vi "MPB_JSON_step editor.vi"() -> ()   [LabVIEW 2020]
uses:
  controls/MPB_step.ctl
  controls/MPB_step_type.ctl
  controls/write_read.ctl
panel:
  out "steps array out":T1[](array[typedef]) {"data num" format="%.3f"}
  in  "read json file":bool
  in  "clear array":bool
  in  "save":bool
  in  "steps array":T1[](array[typedef]) {"data num" format="%.3f"}
  in  "exit":bool
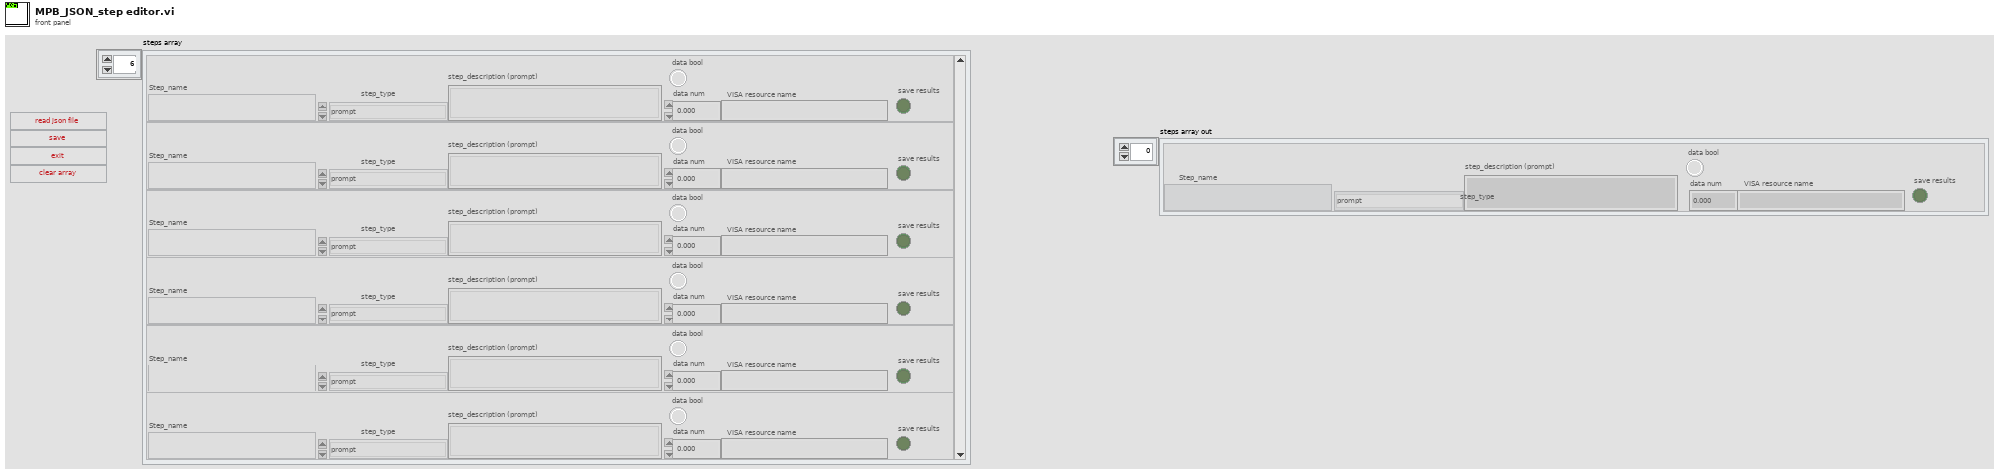
[diagram p1: front panel]
types:
  T1 = typedef "MPB_step.ctl" = cluster{"VISA resource name":string, "data num":dbl, "step_description (prompt)":string, "save results":bool, "step_type":T2, "Step_name":string, "data bool":bool}
  T2 = typedef "MPB_step_type.ctl" = enum16{"default", "prompt", "sequence#", "12V_1_power supply on_off", "12V_2_power supply on_off", "set_hipot_V", "set_hipot_I_limit", "set_hipot_ramping (sec)", "set hipot_hold_time", "read_hipot_V", "read_hipot_I", "set_daq", "read_daq", "flash uds", "wait (sec)", "record_pass_fail", "ac_charge_test", "dc_400V_charging", "HAPS Heater Output", "HAPS Compressor Output", "stop_test", "error_exit"}
  T3 = typedef "write_read.ctl" = enum16{"write", "read"}
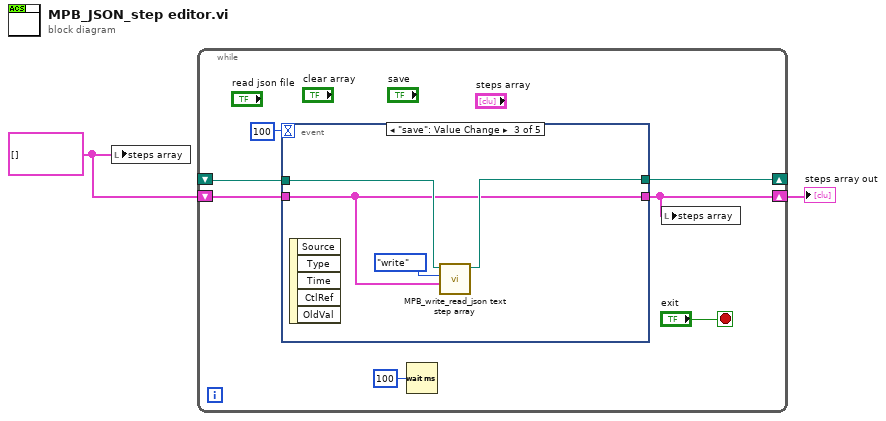
[diagram p0: block diagram]
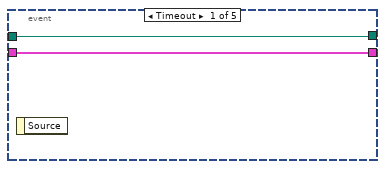
[diagram p2: hidden frame]
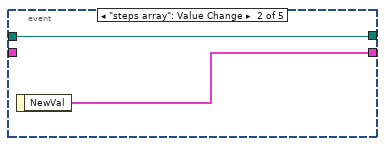
[diagram p3: hidden frame]
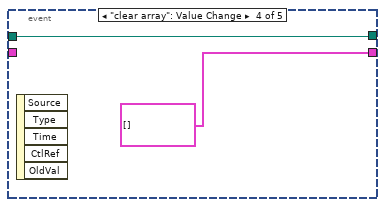
[diagram p4: hidden frame]
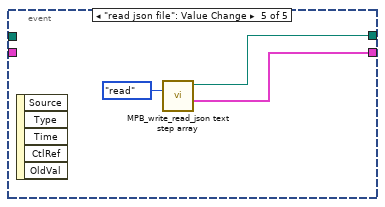
[diagram p5: hidden frame]
diagram:
  w2 = T1[] [] ("steps array out")
  n1 = local write "steps array"(w2) -> ()
  n2 = while {
    shift-right: [w6] -> w1
    shift-left: w2 -> [w8]
    shift-right: [w4] -> _
    shift-left: _ -> [w5]
    stop <- "exit" stop-if-true
    n3 = event shown="[2] \"save\": Value Change" {
      selector: _ -> [_ _ _ _ _]
      dyn-events: _ -> [_ _ _ _ _]
      timeout: 100 -> [_ _ _ _ _]
      tunnel: w8 -> [w11 _ w14 _ _]
      tunnel: [w11 w13 w14 T1[] [] ("steps array out") w21] -> w6
      tunnel: w5 -> [w10 w12 w15 w19 _]
      tunnel: [w10 w12 w16 w19 w20] -> w4
      event Timeout {
        n4 = event-data() -> ()  [unwired: 1 in, 1 out]
      }
      event "steps array": Value Change {
        n5 = event-data() -> ("NewVal"=w13:T1[])  [unwired: 1 in]
      }
      event "save": Value Change {
        n6 = event-data() -> ()  [unwired: 1 in, 5 out]
        n7 = call "MPB_write_read_json text step array.vi"("json_array_from_file"=w14, "write_read"=write_read."write", "File Path"=w15) -> ("File Path"=w16:path)  [unwired: 6 in, 2 out]
      }
      event "clear array": Value Change {
        n8 = event-data() -> ()  [unwired: 1 in, 5 out]
      }
      event "read json file": Value Change {
        n9 = event-data() -> ()  [unwired: 1 in, 5 out]
        n10 = call "MPB_write_read_json text step array.vi"("write_read"=write_read."read") -> ("steps array out"=w21:T1[], "File Path"=w20:path)  [unwired: 8 in, 1 out]
      }
    }
    n11 = Wait (ms)(milliseconds to wait=u32 100) -> ()  [unwired: 1 out]
    n12 = local write "steps array"(w6) -> ()
  }
  "steps array out" <- w1
